vi "NeoPixel Audio Analyzer.vi"(10 "Number Of Elements":i32=192, 11 "Update":bool) -> ()   [LabVIEW 2021]
uses:
  <vilib>/rvi/DataTransferAndStorage/Container/XNode/niFpgaContainer.xnode
  <vilib>/rvi/Memory/Memory_Emulation/niFpgaMemoryEmulationRefIn.vi
  <vilib>/eio/EIONode/EIONode.xnode
  <vilib>/rvi/eio/common/nirviEmuTemplateMethod_errors.vi
  <vilib>/rvi/FIFO/Fifo_Resource/niFpgaFifoEmulationRefIn.vi
  <vilib>/Platform/TimedLoop/XDataNode/wakeup.ctl
  <vilib>/Platform/TimedLoop/XDataNode/XDNodeRunTimeDep.lvlib
  <vilib>/Platform/TimedLoop/XDataNode/nitl_modes.ctl
  <vilib>/Platform/TimedLoop/XDataNode/timing_clust.ctl
  <vilib>/Platform/TimedLoop/XDataNode/XDataNode.xnode
  <vilib>/rvi/interface/RandomDataEmulation/nirviRandomDataFpgaReadWriteTemplate.vi
  <vilib>/rvi/Analysis/measure/FFT/XNode/niFpgaFFT.xnode
  <vilib>/rvi/LocalResourceManager/LocalResourceManager.xnode
  <vilib>/rvi/eio/common/nirviEmuReportErrorAndStop.vi
  <vilib>/rvi/DataTransferAndStorage/Container/Common/niFpgaContainerGetUniqueNameForEmu.vi
  <vilib>/rvi/DataTransferAndStorage/Container/Common/niFpgaContainerSetEmuInfo.vi
  <vilib>/fxp/LVFixedPointQuantizationPolicyTypeDef.ctl
  <vilib>/rvi/Analysis/measure/FFT/simModelSupport/niFpgaFFTSimDfxp.ctl
  <vilib>/rvi/Analysis/measure/FFT/simModelSupport/niFpgaFFTSimArithmeticProperties.ctl
  <vilib>/rvi/Analysis/measure/FFT/simModelSupport/niFPGA FFT Sim Types.ctl
  <vilib>/rvi/Analysis/measure/FFT/simModelSupport/niFPGA FFT Sim Properties.ctl
  <vilib>/rvi/Analysis/measure/FFT/simModelSupport/niFpgaFFTSimModelCore.vi
  Program Files (x86)/National Instruments/LabVIEW 2019/examples/CompactRIO/FPGA Fundamentals/FPGA Math and Analysis/FFT/Type Definitions/Windows.ctl
panel:
  in  "Requested Sample Period (ticks)":u32=1000
  out "Invalid Period":bool
  out "Actual Sample Period (ticks)":u32
  out "Overflow":bool
  in  "Window select":T1=enum."None"
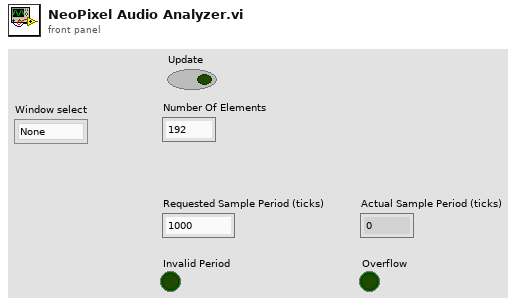
[diagram p1: front panel]
types:
  T1 = typedef "Windows.ctl" = enum16{"Hamming", "Hanning", "None"}
  T2 = typedef "XDNodeRunTimeDep.lvlib/timing_clust.ctl" = cluster{"Expected End [f-1]":u64, "Actual End [f-1]":u64, "Finished Late? [f-1]":bool, "Expected End [i-1]":u64, "Actual End [i-1]":u64, "Finished Late? [i-1]":bool, "Expected Start [i]":u64, "Actual Start [i]":u64, "Expected Start [f]":u64, "Actual Start [f]":u64, "Source Name":string, "Structure Name":string, "Period":i64, "Deadline":i64, "Offset":i64, "Start":i64, "Priority":i32, "Timeout":i32, "Mode":T3, "Wakeup Reason":T4, "Error":errorcluster, "Source Type":string, "Secondary Source Type":string, "Global End Time":u64, "Global Start Time":u64, "Frame Duration":u64, "Iteration Duration":u64, "Assigned CPU":i32, "I/O Scan Engine Mode":u32}
  T3 = typedef "XDNodeRunTimeDep.lvlib/nitl_modes.ctl" = enum32{"No Change", "Process missed periods, maintain original phase", "Discard missed periods, maintain original phase", "Process missed periods, ignore original phase", "Discard missed periods, ignore original phase"}
  T4 = typedef "XDNodeRunTimeDep.lvlib/wakeup.ctl" = enum32{"Normal", "Aborted", "Asynchronous wakeup", "Timing source error", "Timed loop error", "Timeout"}
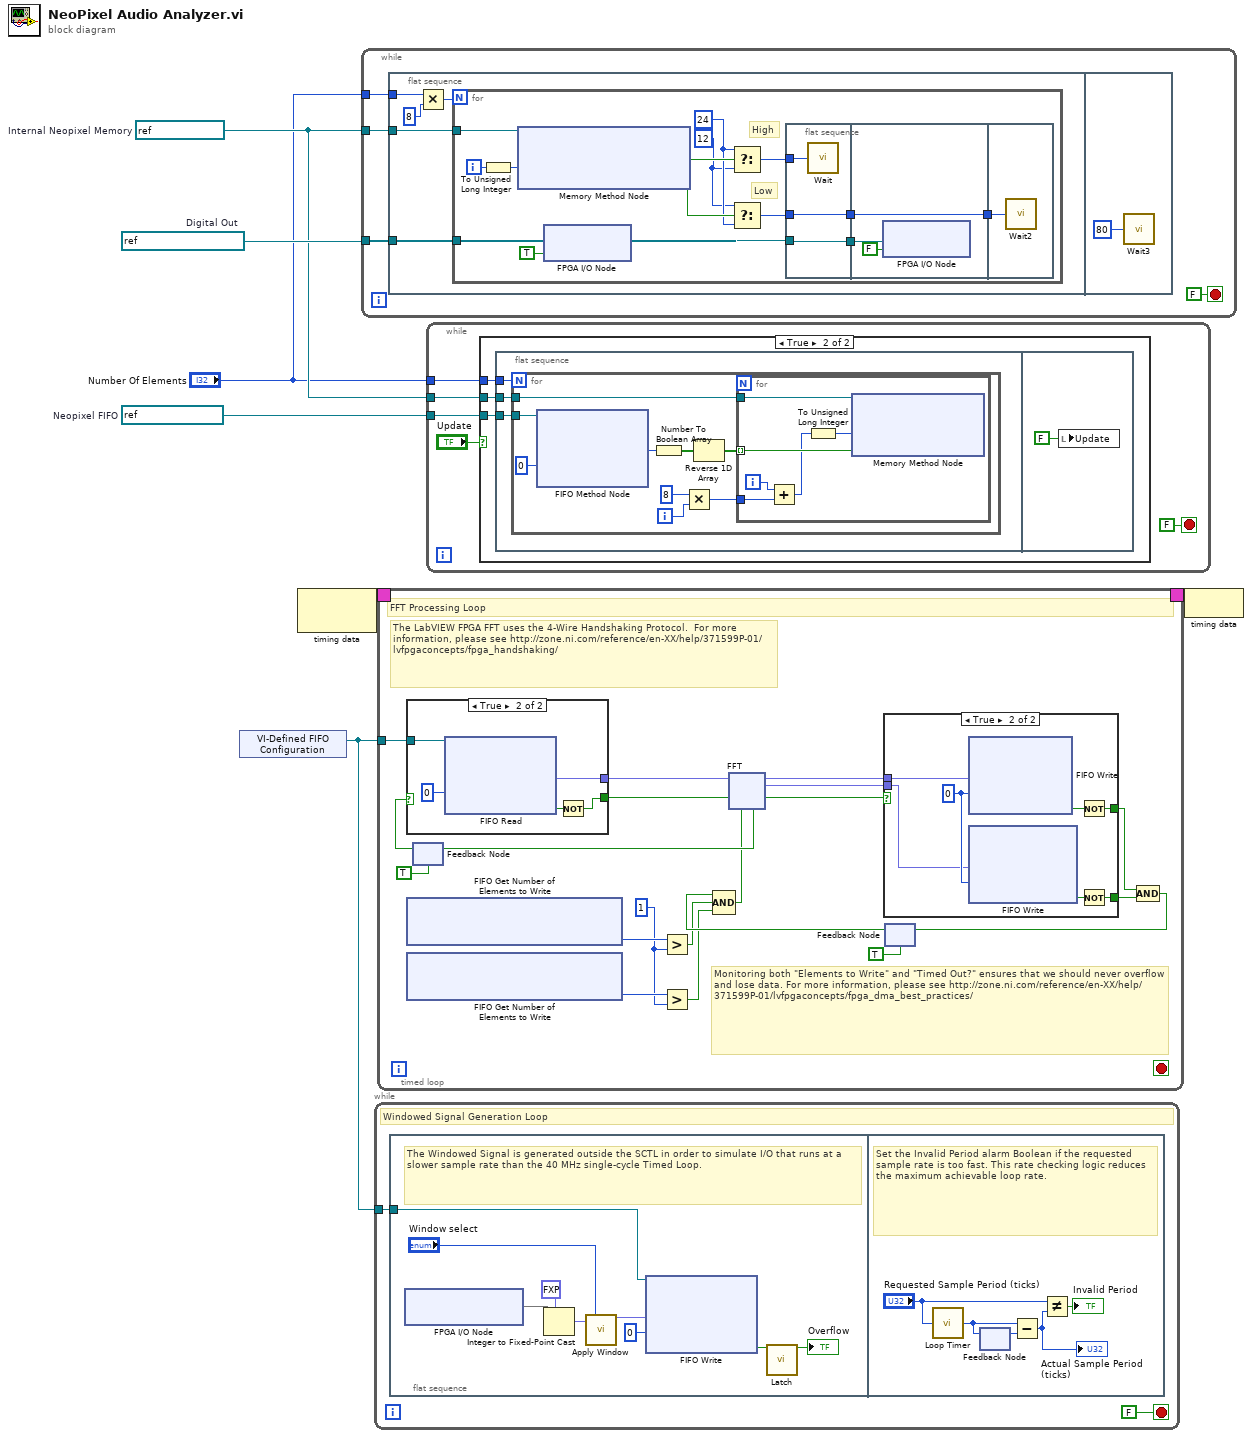
[diagram p0: block diagram]
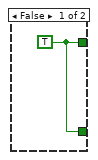
[diagram p2: hidden frame]
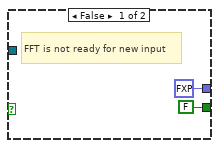
[diagram p3: hidden frame]
diagram:
  w5 = refnum<k21> "Matrix Data"  # Internal Neopixel Memory
  w6 = refnum<k21> "Neopixel FIFO"  # Neopixel FIFO
  w7 = refnum<k21> "ConnectorC/DIO0"  # Digital Out
  n1 = xnode "VI-Defined FIFO Configuration"() -> ("FIFO Out"=w1:refnum<k21>)
  n2 = node-c288() -> (w3:T2)  [unwired: 1 in]
  n3 = while {
    tunnel: w7 -> [w10]
    tunnel: w5 -> [w9]
    tunnel: "Number Of Elements" -> [w8]
    stop <- FALSE stop-if-true
    n4 = flat-sequence {
      tunnel: w10 -> [w16]
      tunnel: w9 -> [w13]
      tunnel: w8 -> [w12]
      frame #0 {
        n5 = Multiply(x=w12, y=8) -> (x*y=w14:i32)
        n6 = for {
          N: w14 -> [_]
          tunnel: w16 -> [w21]
          tunnel: w13 -> [w17]
          i -> [w29]
          w18 = u8 12 ("High False")
          w19 = u8 24 ("High True")
          # "Low"
          # "High"
          n7 = To Unsigned Long Integer(number=w29) -> (unsigned 32bit integer=w30:u32)
          n8 = xnode ("Memory Method Node")("Address"=w30, "Memory In"=w17) -> ("Data"=w26:bool)  [unwired: 1 out]
          n9 = xnode "FPGA I/O Node"("I/O Item"=TRUE, "FPGA I/O In"=w21) -> ("FPGA I/O Out"=w20:refnum<k21>)
          n10 = Select(t=w19, s=w26, f=w18) -> (s? t:f=w27:u8)
          n11 = Select(t=w18, s=w26, f=w19) -> (s? t:f=w25:u8)
          n12 = flat-sequence {
            tunnel: [w32] -> w28
            tunnel: [w33] -> w23
            tunnel: w25 -> [w33]
            tunnel: w27 -> [w31]
            tunnel: w20 -> [w32]
            tunnel: w28 -> [w36]
            tunnel: [w34] -> w24
            tunnel: w23 -> [w34]
            tunnel: w24 -> [w37]
            frame #0 {
              n13 = call "Wait"("Count(Ticks)"=w31) -> ()  [unwired: 1 out]
            }
            frame #1 {
              n14 = xnode "FPGA I/O Node"("I/O Item"=FALSE, "FPGA I/O In"=w36) -> ()  [unwired: 1 out]
            }
            frame #2 {
              n15 = call "Wait2"("Count(Ticks)"=w37) -> ()  [unwired: 1 out]
            }
          }
        }
      }
      frame #1 {
        n16 = call "Wait3"("Count(uSec)"=u16 80 ("Reset (us)")) -> ()  [unwired: 1 out]
      }
    }
  }
  n17 = while {
    tunnel: w1 -> [w40]
    stop <- FALSE stop-if-true
    # "Windowed Signal Generation Loop"
    n18 = flat-sequence {
      tunnel: w40 -> [w46]
      frame #0 {
        # "The Windowed Signal is generated outside the SCTL in order to simulate I/O that runs at a slower sample rate than the 40 MHz single-cycle Timed Loop."
        n19 = xnode "FPGA I/O Node"() -> ("AudioIn/Right"=w43)  [unwired: 1 in, 1 out]
        n20 = Integer to Fixed-Point Cast(fixed-point type=fxp<+/-,16,5> 0.0 ("Signal In"), integer=w43) -> (fixed-point=w41:fxp<+/-,16,5>)
        n21 = call "Apply Window.vi"("Signal In"=w41, "Window select"="Window select") -> ("Windowed Signal Out"=w47:fxp<+/-,16,5>)  [unwired: 13 in]
        n22 = xnode ("FIFO Write")("Element"=w47, "Timeout"=0, "FIFO In"=w46) -> ("Timed Out?"=w45:bool)  [unwired: 1 out]
        n23 = call <vilib>:"Latch.vi"("Input"=w45) -> ("Output"=→"Overflow":bool)  [unwired: 14 in]
      }
      frame #1 {
        # "Set the Invalid Period alarm Boolean if the requested sample rate is too fast. This rate checking logic reduces the maximum achievable loop rate."
        n24 = call "Loop Timer"("Count(Ticks)"="Requested Sample Period (ticks)") -> ("Tick Count(Ticks)"=w50:u32)
        n25 = feedback #1() -> (w51:u32)  [unwired: 1 in]
        n26 = feedback-in #1(w50) -> ()
        n27 = Subtract(x=w50, y=w51) -> (x-y=w54:u32)
        "Actual Sample Period (ticks)" <- w54
        n28 = Not Equal?(x="Requested Sample Period (ticks)", y=w54) -> (x != y?=→"Invalid Period":bool)
      }
    }
  }
  n29 = timed-loop {
    timing: w3 -> [_]
    timing-out: [_] -> w2
    tunnel: w1 -> [w70]
    stop <- _ stop-if-true
    w60 = u32 1 ("y")
    # "Monitoring both \"Elements to Write\" and \"Timed Out?\" ensures that we should never overflow and lose data. For more information, please see http://zone.ni.com/reference/en-XX/help/371599P-01/lvfpgaconcepts/fpga_dma_best_practices/"
    # "The LabVIEW FPGA FFT uses the 4-Wire Handshaking Protocol.  For more information, please see http://zone.ni.com/reference/en-XX/help/371599P-01/lvfpgaconcepts/fpga_handshaking/"
    # "FFT Processing Loop"
    n30 = xnode ("FIFO Get Number of Elements to Write")() -> ("Number of Elements to Write"=w62:u32)  [unwired: 1 in, 1 out]
    n31 = xnode ("FIFO Get Number of Elements to Write")() -> ("Number of Elements to Write"=w61:u32)  [unwired: 1 in, 1 out]
    n32 = feedback #2(TRUE ("ready for input")) -> (w74:bool)
    n33 = case shown="True" w74 {
      tunnel: [FALSE w114] -> w71
      tunnel: [fxp<+/-,16,5> 0.0 ("Element") w115] -> w73
      tunnel: w70 -> [_ w111]
      frame False {
        # "FFT is not ready for new input"
      }
      frame True {
        n34 = xnode ("FIFO Read")("Timeout"=0, "FIFO In"=w111) -> ("Element"=w115:fxp<+/-,16,5>, "Timed Out?"=w113:bool)  [unwired: 1 out]
        n35 = Not(x=w113) -> (.not. x?=w114:bool)
      }
    }
    n36 = Greater?(x=w62, y=w60) -> (0:w57:bool)
    n37 = Greater?(x=w61, y=w60) -> (0:w56:bool)
    n38 = feedback #3(TRUE) -> (w58:bool)
    n39 = Compound Arithmetic op=AND(w58, w57, w56) -> (w59:bool)
    n40 = xnode "FFT"("real data in"=w73, "input valid"=w71, "ready for output"=w59) -> ("ready for input"=w72:bool, "real data out"=w69:fxp<+/-,25,14>, "imaginary data out"=w68:fxp<+/-,25,14>, "output valid"=w67:bool)  [unwired: 2 in, 1 out]
    n41 = feedback-in #2(w72) -> ()
    n42 = case shown="True" w67 {
      tunnel: w69 -> [_ w103]
      tunnel: w68 -> [_ w102]
      tunnel: [w101 w105] -> w66
      tunnel: [w101 w104] -> w65
      frame False {
        w101 = TRUE ("Timed Out?")
      }
      frame True {
        w108 = 0 ("Timeout")
        n43 = xnode ("FIFO Write")("Element"=w103, "Timeout"=w108) -> ("Timed Out?"=w107:bool)  [unwired: 1 in, 1 out]
        n44 = xnode ("FIFO Write")("Element"=w102, "Timeout"=w108) -> ("Timed Out?"=w106:bool)  [unwired: 1 in, 1 out]
        n45 = Not(x=w107) -> (.not. x?=w105:bool)
        n46 = Not(x=w106) -> (.not. x?=w104:bool)
      }
    }
    n47 = Compound Arithmetic op=AND(w66, w65) -> (w64:bool)
    n48 = feedback-in #3(w64) -> ()
  }
  n49 = while {
    tunnel: w6 -> [w120]
    tunnel: w5 -> [w119]
    tunnel: "Number Of Elements" -> [w118]
    stop <- FALSE stop-if-true
    n50 = case shown="True" "Update" {
      tunnel: w120 -> [_ w125]
      tunnel: w119 -> [_ w124]
      tunnel: w118 -> [_ w123]
      frame False {
      }
      frame True {
        n51 = flat-sequence {
          tunnel: w125 -> [w128]
          tunnel: w124 -> [w127]
          tunnel: w123 -> [w126]
          frame #0 {
            n52 = for {
              N: w126 -> [_]
              tunnel: w128 -> [w131]
              tunnel: w127 -> [w129]
              i -> [w137]
              n53 = xnode ("FIFO Method Node")("Timeout"=0, "FIFO In"=w131) -> ("Element"=w132:u8)  [unwired: 2 out]
              n54 = Number To Boolean Array(number=w132) -> (Boolean array=w134:bool[])
              n55 = Multiply(x=8, y=w137) -> (x*y=w135:i32)
              n56 = Reverse 1D Array(array=w134) -> (reversed array=w133:bool[])
              n57 = for {
                tunnel: w133 -> [w142] mode=indexing
                tunnel: w135 -> [w140]
                tunnel: w129 -> [w138]
                i -> [w141]
                n58 = Add(x=w141, y=w140) -> (x+y=w139:i32)
                n59 = To Unsigned Long Integer(number=w139) -> (unsigned 32bit integer=w143:u32)
                n60 = xnode ("Memory Method Node")("Address"=w143, "Data"=w142, "Memory In"=w138) -> ()  [unwired: 1 out]
              }
            }
          }
          frame #1 {
            n61 = local write "Update"(FALSE ("Update")) -> ()
          }
        }
      }
    }
  }
  n62 = node-c288(w2) -> ()
